vi "setUp.vi"(8 "error in (no error)":errorcluster, 11 "reference in":refnum<class "Test Network Stream Initiator Connect.lvclass">) -> (0 "error out":errorcluster, 3 "reference out":refnum<class "Test Network Stream Initiator Connect.lvclass">)   [LabVIEW 2020, in "Test Network Stream Initiator Connect.lvclass"]
doc: "setUp runs prior to the test method during test execution. Use this method to initialize any object data required by your tests."
uses:
  Test Network Stream Initiator Connect.lvclass
  <vilib>/addons/_JKI Toolkits/VI Tester/TestCase.llb/TestCase.lvclass
  Source/Protocols/Network Stream Strategy/Network Stream Initiator/Network Stream Initiator.lvclass
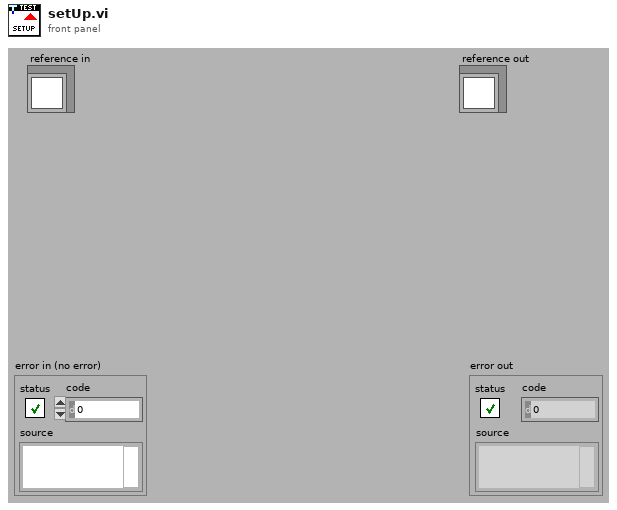
[diagram p1: front panel]
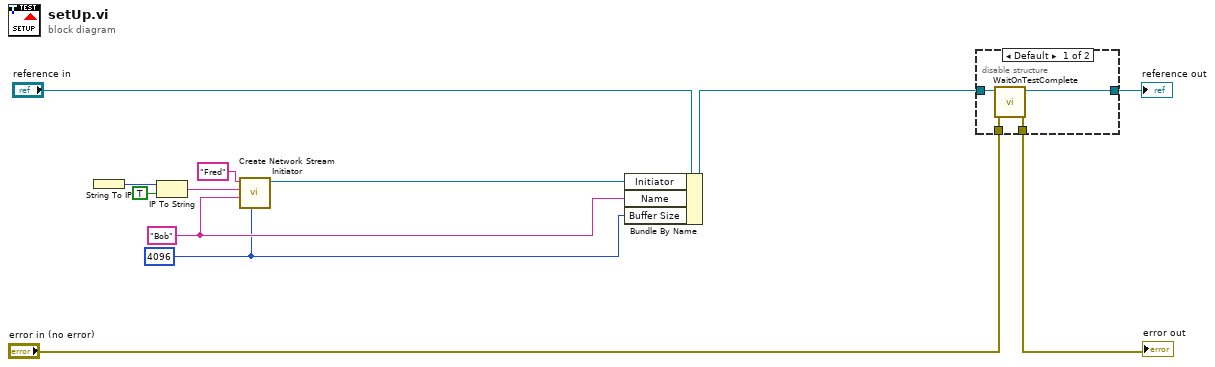
[diagram p0: block diagram]
diagram:
  w1 = 4096 ("Buffer Size")
  w4 = "Bob" ("Remote Name")
  n1 = String To IP() -> (0:w7:u32)  [unwired: 1 in]
  n2 = IP To String(1:TRUE ("dot notation? (F)"), 2:w7) -> (0:w3:string)
  n3 = call "Create Network Stream Initiator.vi"("Buffer Size"=w1, "Remote Name"=w4, "Remote Address"=w3, "Name"="Fred") -> ("Network Stream Initiator out"=w5:refnum<class "Network Stream Initiator.lvclass">)  [unwired: 7 in]
  n4 = Bundle By Name(cluster="reference in", "Initiator"=w5, "Name"=w4, "Buffer Size"=w1) -> (w8:refnum<class "Test Network Stream Initiator Connect.lvclass">)
  n5 = disable-structure shown="Default" {
    disable-tunnel: "error in (no error)" -> [w16 w17]
    disable-tunnel: [w15 w17] -> w11
    disable-tunnel: [w14 w18] -> w9
    disable-tunnel: w8 -> [w13 w18]
    frame condition #0 (active) {
      n6 = call <vilib>:"WaitOnTestComplete.vi"("error in (no error)"=w16, "TestCase in"=w13) -> ("error out"=w15:errorcluster, "TestCase out"=w14:refnum<class "Test Network Stream Initiator Connect.lvclass">)  [unwired: 8 in]
    }
    frame condition #1 {
    }
  }
  "error out" <- w11
  "reference out" <- w9
